vi "From JSON Tree.vi"(8 "error in (no error)":errorcluster, 10 "JSON in":refnum<class "JSON Datatype.lvclass">, 11 "result in":refnum<class "result.lvclass">) -> (0 "error out":errorcluster, 3 "result out":refnum<class "result.lvclass">)   [LabVIEW 2015, in "result.lvclass"]
uses:
  result.lvclass
  <vilib>/National Instruments/JSON Support for LabVIEW/JSON Data Classes/JSON Datatype/JSON Datatype.lvclass
  result.lvclass/result.ctl
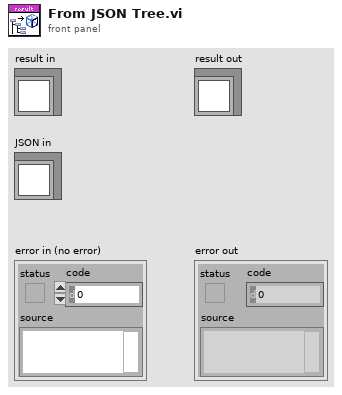
[diagram p1: front panel]
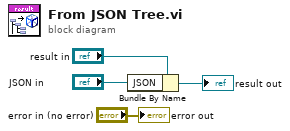
[diagram p0: block diagram]
diagram:
  n1 = Bundle By Name(cluster="result in", "JSON"="JSON in") -> (→"result out":refnum<class "result.lvclass">)
  "error out" <- "error in (no error)"
